vi "list_packages.vi"(8 "error in (no error)":errorcluster, 10 "package_manager":string="nipm", 11 "dragon_file_path":path=path "C:/Projects/labview-project-load-tools/rust_src/toml_edit_dll/lv_src/test.toml") -> ()   [LabVIEW 2020]
uses:
  dragon_toml_64.dll
panel:
  out "packages":string[](array[string])
  out "error out":errorcluster
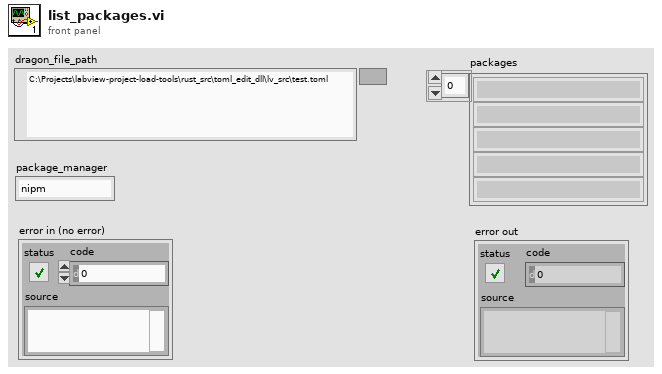
[diagram p1: front panel]
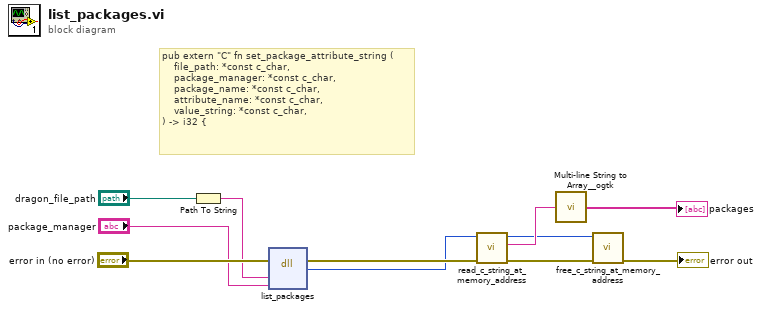
[diagram p0: block diagram]
diagram:
  # "pub extern \"C\" fn set_package_attribute_string (\n    file_path: *const c_char,\n    package_manager: *const c_char,\n    package_name: *const c_char,\n    attribute_name: *const c_char,\n    value_string: *const c_char,\n) -> i32 {"
  n1 = Path To String(path="dragon_file_path") -> (string=w8:string)
  n2 = dll-call lib="C:/Projects/labview-project-load-tools/rust_src/toml_edit_dll/lv_src/dragon_toml_*.dll" fn="list_packages"(error in="error in (no error)", "file_path"=w8, "package_manager"="package_manager") -> (error out=w5:errorcluster, "result"=w2:u64)  [unwired: 4 in, 1 out]
  n3 = call "read_c_string_at_memory_address.vi"("error in (no error)"=w5, "memory_address"=w2) -> ("error out"=w7:errorcluster, "string"=w3:string, "memory_address out"=w1:u64)  [unwired: 7 in]
  n4 = call <userlib>:"Multi-line String to Array__ogtk.vi"("string"=w3) -> ("lines"=→"packages":string[])
  n5 = call "free_c_string_at_memory_address.vi"("error in (no error)"=w7, "memory_address"=w1) -> ("error out"=→"error out":errorcluster)  [unwired: 9 in]
